vi "Write UI object.vi"(8 "error in (no error)":errorcluster, 10 "Mag Lab Measure Interface.lvclass":refnum<class "Mag Lab Measure UI.lvclass">, 11 "Mag Lab Measure Base in":refnum<class "Mag Lab Measure Base.lvclass">) -> (0 "error out":errorcluster, 3 "Mag Lab Measure Base out":refnum<class "Mag Lab Measure Base.lvclass">)   [LabVIEW 2015, in "Mag Lab Measure Base.lvclass"]
uses:
  Mag Lab Measure Base.lvclass
  Mag Lab Measure Interface/Mag Lab Measure UI.lvclass
  Mag Lab Measure Base.lvclass/Mag Lab Measure Base.ctl
  Mag Lab Root/Mag Lab Root.lvclass/Mag Lab Root.ctl
  Mag Lab Root/Mag Lab Root.lvclass
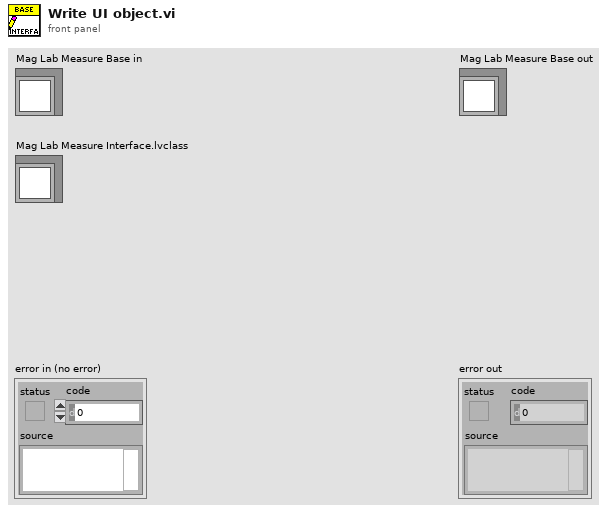
[diagram p1: front panel]
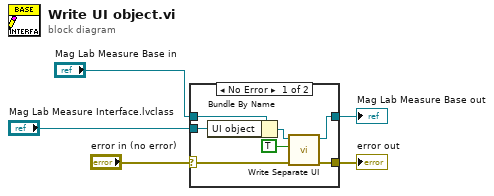
[diagram p0: block diagram]
diagram:
  n1 = case shown="No Error" "error in (no error)" {
    selector: "error in (no error)" -> [w8 w13]
    tunnel: [w7 w13] -> w4
    tunnel: [w9 w14] -> w2
    tunnel: "Mag Lab Measure Base in" -> [w12 w14]
    tunnel: "Mag Lab Measure Interface.lvclass" -> [w11 _]
    frame No Error {
      n2 = Bundle By Name(cluster=w12, "UI object"=w11) -> (w10:refnum<class "Mag Lab Measure Base.lvclass">)
      n3 = call "Write Separate UI.vi"("error in (no error)"=w8, "Separate UI"=TRUE, "Mag Lab Root in"=w10) -> ("error out"=w7:errorcluster, "Mag Lab Root out"=w9:refnum<class "Mag Lab Measure Base.lvclass">)  [unwired: 7 in]
    }
    frame Error {
    }
  }
  "error out" <- w4
  "Mag Lab Measure Base out" <- w2
